vi "FL_Get_Run_Bout_and_Time.vi"(0 "Speed, mm/s":dbl format="%#_13g", 1 "Run Lengts distribution array in":u32[](array[numeric]), 3 "Speed lower threshold, mm/s":dbl=8.0 format="%#_13g", 4 "Run times distribution array in":u32[](array[numeric]), 5 "Run Lengths bin array":dbl[](array[numeric]), 8 "Run times bin array":dbl[](array[numeric])) -> (6 "Run Lengts distribution array out":u32[](array[numeric]), 9 "Run times distribution array out":u32[](array[numeric]))   [LabVIEW 2016]
panel:
  out "Run time, s":dbl
  out "Run Length, m":dbl
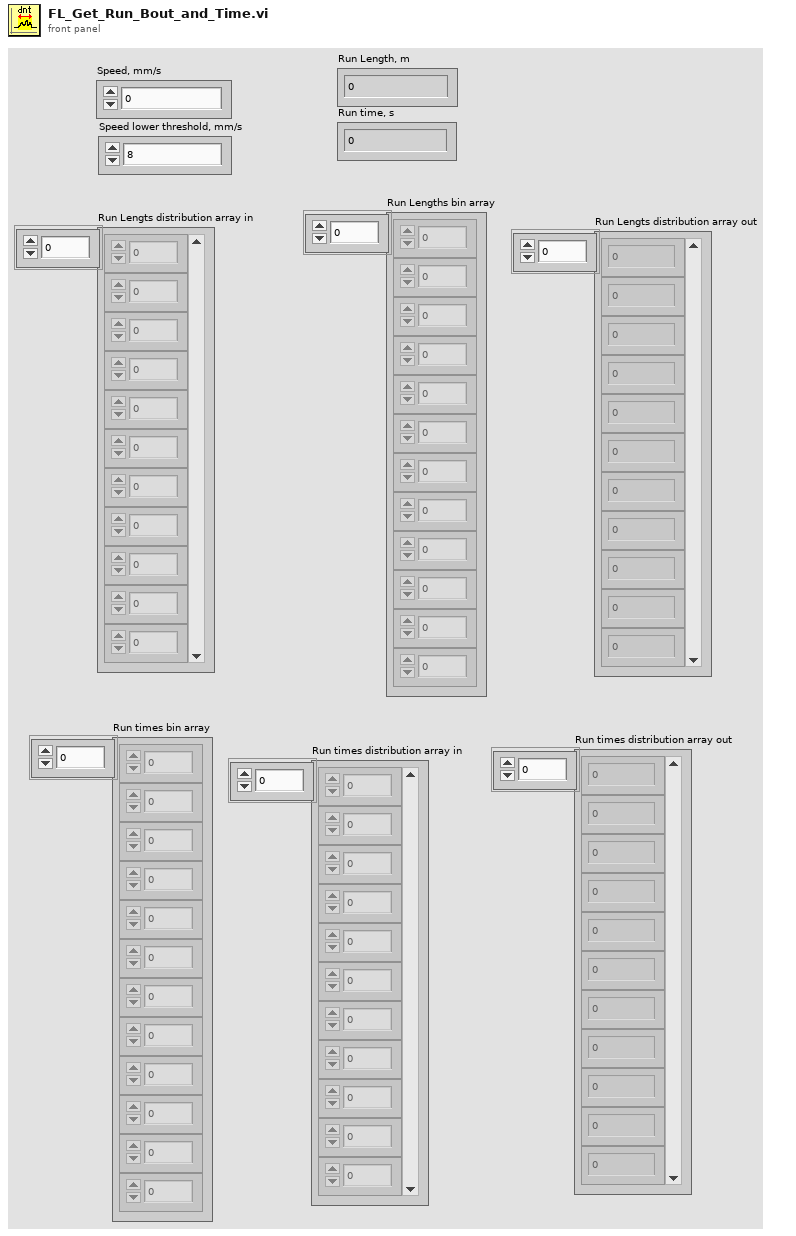
[diagram p1: front panel]
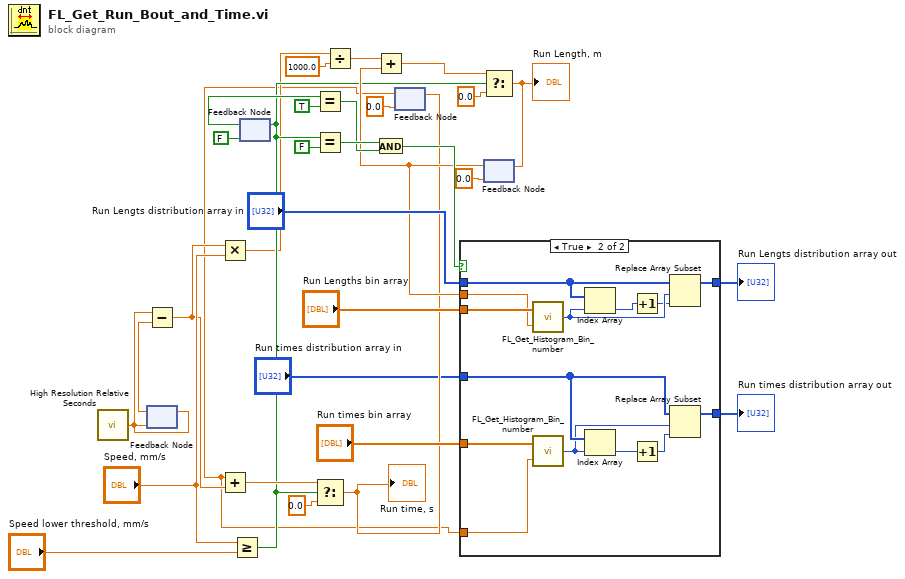
[diagram p0: block diagram]
diagram:
  n1 = call <vilib>:"High Resolution Relative Seconds.vi"() -> ("relative seconds"=w26:dbl)
  n2 = feedback #1(w26) -> (w30:dbl)
  n3 = Subtract(x=w26, y=w30) -> (x-y=w5:dbl)
  n4 = feedback-in #1(w26) -> ()
  n5 = Multiply(x=w5, y="Speed, mm/s") -> (x*y=w3:dbl)
  n6 = Greater Or Equal?(x="Speed, mm/s", y="Speed lower threshold, mm/s") -> (x >= y?=w10:bool)
  n7 = feedback-in #2(w10) -> ()
  n8 = feedback #2(FALSE) -> (w23:bool)
  n9 = Equal?(x=w23, y=TRUE) -> (x = y?=w20:bool)
  n10 = Equal?(x=w10, y=FALSE) -> (x = y?=w21:bool)
  n11 = Divide(x=w3, y=1000.0) -> (x/y=w4:dbl)
  n12 = And(x=w21, y=w20) -> (x .and. y?=w15:bool)
  n13 = feedback #3(0.0) -> (w1:dbl)
  n14 = Add(x=w1, y=w5) -> (x+y=w12:dbl)
  n15 = Select(t=w12, s=w10, f=0.0) -> (s? t:f=w8:dbl)
  "Run time, s" <- w8
  n16 = feedback-in #3(w8) -> ()
  n17 = feedback #4(0.0) -> (w14:dbl)
  n18 = Add(x=w4, y=w14) -> (x+y=w28:dbl)
  n19 = case shown="True" w15 {
    tunnel: "Run Lengts distribution array in" -> [w34 w45]
    tunnel: "Run Lengths bin array" -> [_ w44]
    tunnel: w14 -> [_ w43]
    tunnel: [w34 w42] -> w16
    tunnel: "Run times bin array" -> [_ w41]
    tunnel: w1 -> [_ w40]
    tunnel: "Run times distribution array in" -> [w33 w36]
    tunnel: [w33 w37] -> w6
    frame False {
    }
    frame True {
      n20 = call "FL_Get_Histogram_Bin_number.vi"("Current value"=w43, "Bins array"=w44) -> ("Bin assignment"=w47:i32)
      n21 = call "FL_Get_Histogram_Bin_number.vi"("Current value"=w40, "Bins array"=w41) -> ("Bin assignment"=w35:i32)
      n22 = Index Array(array=w45, index=w47) -> (element=w48:u32)
      n23 = Index Array(array=w36, index=w35) -> (element=w38:u32)
      n24 = Increment(x=w48) -> (x+1=w46:u32)
      n25 = Increment(x=w38) -> (x+1=w39:u32)
      n26 = Replace Array Subset(array=w45, new element=w46, index=w47) -> (w42:u32[])
      n27 = Replace Array Subset(array=w36, new element=w39, index=w35) -> (w37:u32[])
    }
  }
  "Run Lengts distribution array out" <- w16
  "Run times distribution array out" <- w6
  n28 = Select(t=w28, s=w10, f=0.0) -> (s? t:f=w17:dbl)
  "Run Length, m" <- w17
  n29 = feedback-in #4(w17) -> ()
